vi "LinearSystemSim_Execute.vi"(5 "Linear System":T1, 6 "dT_Seconds":dbl=0.02, 7 "Measurement Std Dev":dbl[](array[numeric]), 9 "Battery Voltage":dbl=12.0, 10 "Demand Array (CO)":dbl[](array[numeric]), 11 "Initial States":dbl[](array[numeric])) -> (0 "Error":bool, 3 "Outputs":dbl[](array[numeric]), 4 "out LinearSystemSim":T3)   [LabVIEW 2019, in "Trajectory_Library.lvlib"]
doc: "Single call LabVIEW function to simulate a linear system. \n\n\nInputs:\n - Linear System -- Linear System -- The linear system to be simulted.\n - Measurement Std Dev -- double array (outputs) -- Optional, siulation output standard deviations (Default: 0.0)\n - Initial States -- double array (states) -- Optional, contains initial state values. (Default: contents of linear system)\n - Demand Array (CO) -- double array(inputs) -- demand values. (+/- 1.0 ) These are turned into voltages by multiplying by the battery voltage.\n - Battery Voltage -- double -- Optional, current simulated battery voltage (Volts Default: 12.0)\n - dT Sec -- double -- Optional,, update period (Seconds, Default: 0.02)\n\nOutputs:\n - Outputs -- double array (outputs) -- Current system outputs.\n - Error -- boolean -- If TRUE an error occured.\n - outLinearSystemSim -- cluster -- Current internal data cluster."
uses:
  Trajectory_Library.lvlib
  TypeDef/LINEAR_SYSTEM_SIM.ctl
  TypeDef/LINEAR_SYSTEM.ctl
  <vilib>/Analysis/Matrix/Datatypes/RealMatrix.ctl
  <vilib>/Analysis/Matrix/Numeric/Conversions/Array To Matrix - RA.vi
  <vilib>/Analysis/Matrix/Numeric/Conversions/Matrix To Array - RM.vi
  <vilib>/Analysis/Matrix/NI_Matrix.lvlib
panel:
  # "<States,States>"
  # "<States,Inputs>"
  # "<Outputs,States>"
  # "<Outputs,Inputs>"
  # "<States, 1>"
  # "<Outputs, 1>"
  # "<Inputs, 1>"
  # "<Outputs, 1>"
  # "<States,States>"
  # "<States,Inputs>"
  # "<Outputs,States>"
  # "<Outputs,Inputs>"
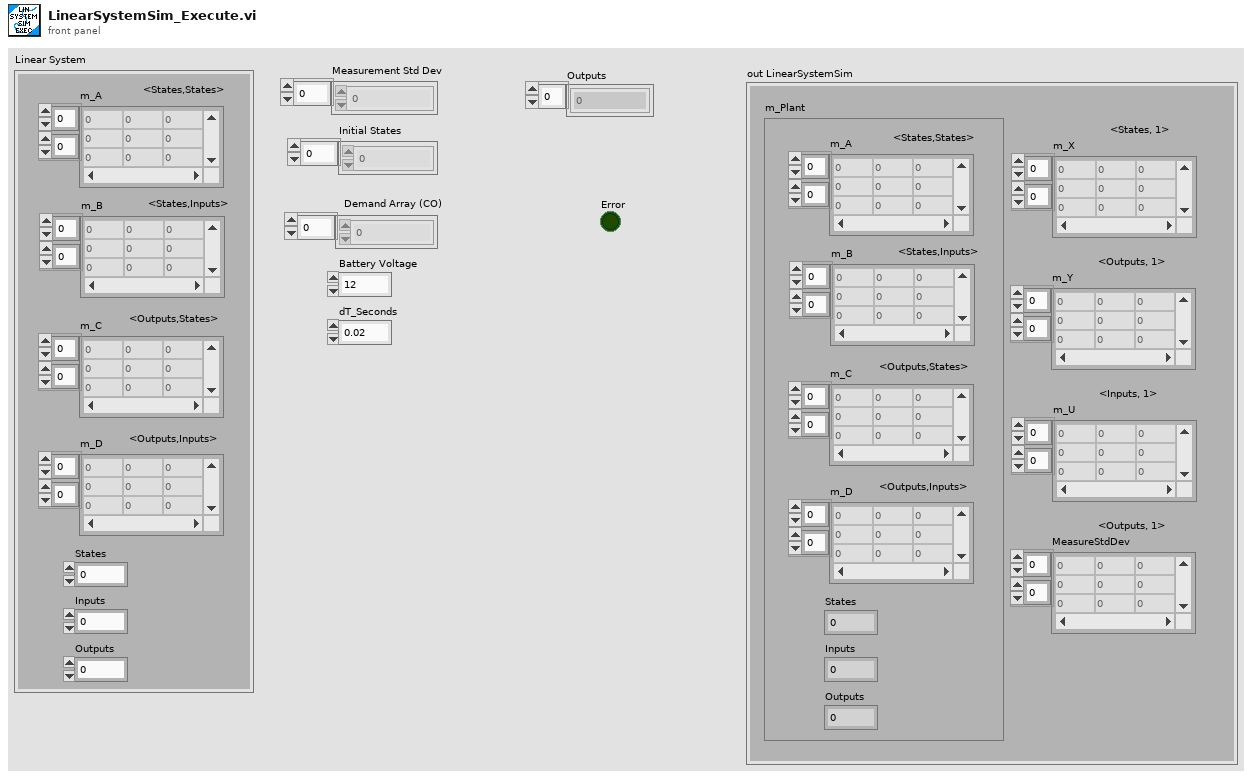
[diagram p1: front panel]
types:
  T1 = typedef "Trajectory_Library.lvlib/LINEAR_SYSTEM.ctl" = cluster{"m_A":T2, "m_B":T2, "m_C":T2, "m_D":T2, "States":i32, "Inputs":i32, "Outputs":i32}
  T2 = typedef "NI_Matrix.lvlib/RealMatrix.ctl" = dbl[][]
  T3 = typedef "Trajectory_Library.lvlib/LINEAR_SYSTEM_SIM.ctl" = cluster{"m_Plant":T1, "m_X":T2, "m_Y":T2, "m_U":T2, "MeasureStdDev":T2}
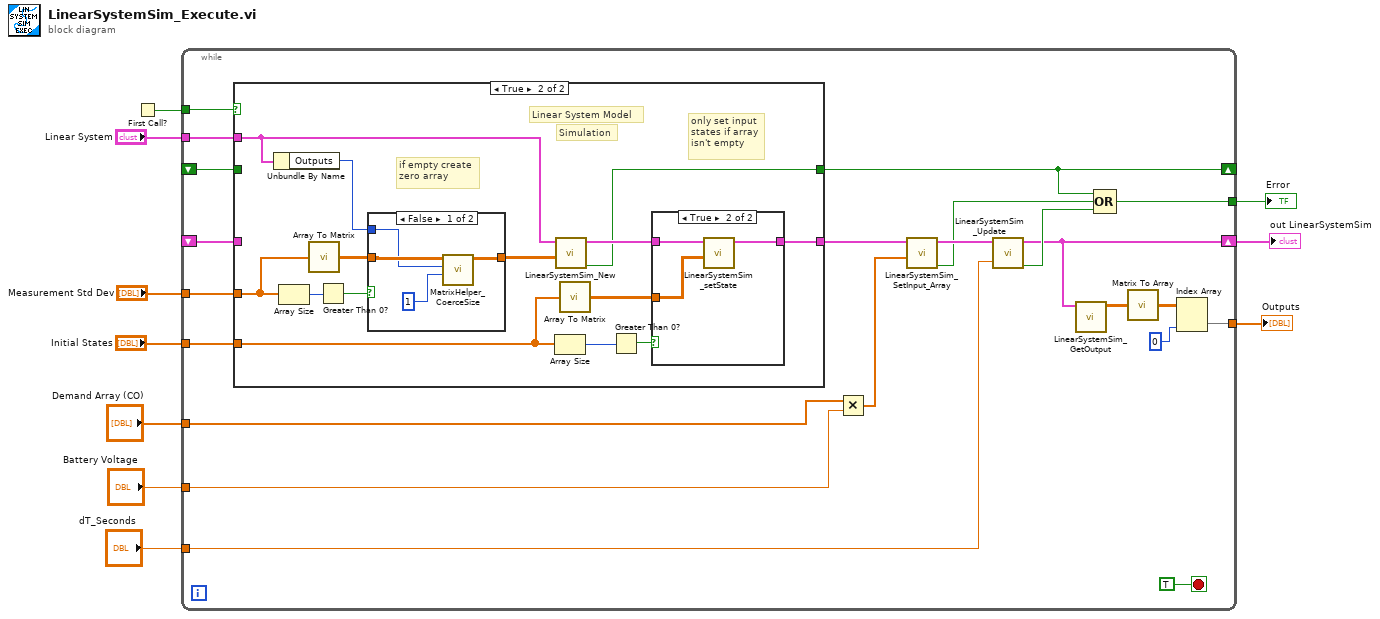
[diagram p0: block diagram]
diagram:
  n1 = First Call?() -> (First Call?: T/F=w7:bool)
  n2 = while {
    tunnel: "Demand Array (CO)" -> [w32]
    tunnel: "Battery Voltage" -> [w31]
    tunnel: "dT_Seconds" -> [w30]
    shift-right: [w16] -> w1
    shift-left: _ -> [w27]
    tunnel: w7 -> [w28]
    tunnel: "Linear System" -> [w26]
    shift-right: [w18] -> _
    shift-left: _ -> [w24]
    tunnel: [w22] -> w5
    tunnel: "Measurement Std Dev" -> [w21]
    tunnel: "Initial States" -> [w15]
    tunnel: [w11] -> w2
    stop <- TRUE stop-if-true
    n3 = case shown="True" w28 {
      tunnel: w27 -> [w33 _]
      tunnel: [w33 w43] -> w20
      tunnel: w26 -> [_ w36]
      tunnel: [w34 w42] -> w18
      tunnel: w24 -> [w34 _]
      tunnel: w21 -> [_ w40]
      tunnel: w15 -> [_ w47]
      frame False {
      }
      frame True {
        # "if empty create\nzero array"
        # "only set input\nstates if array\nisn't empty"
        # "Simulation"
        # "Linear System Model"
        n4 = Unbundle By Name(w36) -> ("Outputs"=w35:i32)
        n5 = Array Size(array=w40) -> (size(s)=w41:i32)
        n6 = call-poly <vilib>:"Array To Matrix.vi"("Real 1D Array"=w40) -> ("Real Matrix (Column Vector)"=w38:T2)
        n7 = Greater Than 0?(x=w41) -> (x > 0?=w39:bool)
        n8 = case shown="False" w39 {
          tunnel: w38 -> [w51 w53]
          tunnel: [w52 w53] -> w37
          tunnel: w35 -> [w49 _]
          frame False {
            n9 = call "MatrixHelper_CoerceSize.vi"("Columns"=1, "Rows"=w49, "input matrix"=w51) -> ("output matrix"=w52:T2)  [unwired: 7 in, 1 out]
          }
          frame True {
          }
        }
        n10 = Array Size(array=w47) -> (size(s)=w46:i32)
        n11 = call "LinearSystemSim_New.vi"("MeasurementStdDev"=w37, "System"=w36) -> ("Size Coerced"=w42:bool, "LinearSystemSim"=w44:T3)  [unwired: 8 in]
        n12 = call-poly <vilib>:"Array To Matrix.vi"("Real 1D Array"=w47) -> ("Real Matrix (Column Vector)"=w48:T2)
        n13 = Greater Than 0?(x=w46) -> (x > 0?=w45:bool)
        n14 = case shown="True" w45 {
          tunnel: w48 -> [_ w55]
          tunnel: w44 -> [w54 w57]
          tunnel: [w54 w56] -> w43
          frame False {
          }
          frame True {
            n15 = call "LinearSystemSim_setState.vi"("System State"=w55, "in LinearSystemSim"=w57) -> ("out LinearSystemSim"=w56:T3)  [unwired: 8 in, 1 out]
          }
        }
      }
    }
    n16 = Multiply(x=w32, y=w31) -> (x*y=w19:dbl[])
    n17 = call "LinearSystemSim_SetInput_Array.vi"("Input"=w19, "in LinearSystemSim"=w20) -> ("Size Coerced"=w17:bool, "out LinearSystemSim"=w29:T3)  [unwired: 8 in]
    n18 = call "LinearSystemSim_Update.vi"("dT_Seconds"=w30, "in LinearSystemSim"=w29) -> ("Error"=w23:bool, "out LinearSystemSim"=w16:T3)  [unwired: 8 in]
    n19 = call "LinearSystemSim_GetOutput.vi"("LinearSysemSim"=w16) -> ("Output"=w14:T2)  [unwired: 10 in]
    n20 = Compound Arithmetic op=OR(w18, w17, w23) -> (w22:bool)
    n21 = call-poly <vilib>:"Matrix To Array.vi"("Real Matrix"=w14) -> ("Real 2D Array"=w13:dbl[][])
    n22 = Index Array(array=w13, index (col)=0 ("disabled index (col)")) -> (element=w11:dbl[])  [unwired: 1 in]
  }
  "out LinearSystemSim" <- w1
  "Error" <- w5
  "Outputs" <- w2
